vi "files_path.vi"(5 "Path":path) -> (0 "file name":string, 1 "files path":path)   [LabVIEW 2010]
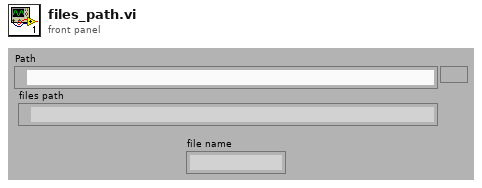
[diagram p1: front panel]
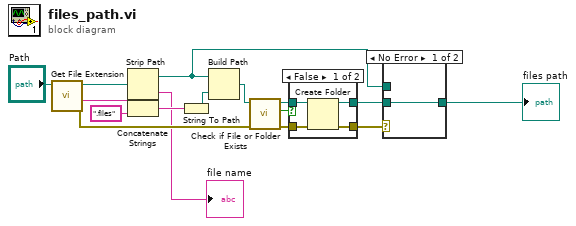
[diagram p0: block diagram]
diagram:
  n1 = call <vilib>:"Get File Extension.vi"("file"="Path") -> ("error out"=w10:errorcluster, "filename without extension"=w4:string, "dup file"=w8:path)  [unwired: 7 in, 1 out]
  n2 = Strip Path(path=w8) -> (stripped path=w3:path, name=→"file name":string)
  n3 = Concatenate Strings(w4, ".files" ("string")) -> (w14:string)
  n4 = String To Path(string=w14) -> (path=w15:path)
  n5 = Build Path(base path=w3, name or relative path=w15) -> (appended path=w9:path)
  n6 = call <vilib>:"Check if File or Folder Exists.vi"("error in (no error)"=w10, "path"=w9) -> ("error out"=w12:errorcluster, "file or folder exists?"=w11:bool, "dup path"=w13:path)  [unwired: 7 in]
  n7 = case shown="False" w11 {
    tunnel: [w20 w21] -> w6
    tunnel: [w19 w22] -> w7
    tunnel: w12 -> [w18 w21]
    tunnel: w13 -> [w17 w22]
    frame False {
      n8 = Create Folder(path (use dialog)=w17, error in=w18) -> (created path=w19:path, error out=w20:errorcluster)  [unwired: 1 in, 1 out]
    }
    frame True {
    }
  }
  n9 = case shown="No Error" w6 {
    tunnel: [w23 w24] -> w2
    tunnel: w7 -> [w23 _]
    tunnel: w3 -> [_ w24]
    frame No Error {
    }
    frame Error {
    }
  }
  "files path" <- w2
